vi "BuildUI.vi"(8 "error in (no error)":errorcluster, 11 "reference in":refnum<class "ProjectBuilder.lvclass">) -> (0 "error out":errorcluster, 3 "reference out":refnum<class "ProjectBuilder.lvclass">)   [LabVIEW 2015, in "ProjectBuilder.lvclass"]
uses:
  ProjectBuilder.lvclass
  BrowerTree/Type Definition/Symbol Index.ctl
  Product/Interface/Type Definition/BuildUI Workflow.ctl
  ProjectBuilder.lvclass/ProjectBuilder.ctl
  <vilib>/Utility/error.llb/Error Cluster From Error Code.vi
  <vilib>/ErrorRing/Error Ring.xnode
  Product/Interface/Part.lvclass
  AbstractBuilder/AbstractBuilder.lvclass
  BrowerTree/BrowerTree.lvclass
panel:
  in  "Previous":bool
  in  "Next":bool
  in  "Cancel":bool
  in  "SymbolIndex":T1
  in  "ComponentName":string caption="Name"
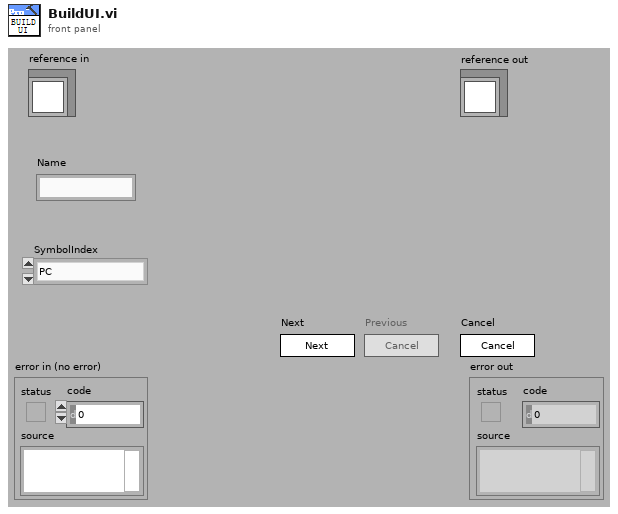
[diagram p1: front panel]
types:
  T1 = typedef "BrowerTree.lvclass/Symbol Index.ctl" = enum16{"PC", "Project", "Module", "DebugTask", "Communication"}
  T2 = typedef "AbstractBuilder.lvclass/BuildUI Workflow.ctl" = enum16{"Init", "Work", "Finish"}
  T3 = enum8{"Enabled", "Disabled", "Disabled and Grayed Out"}
  T4 = enum32{"Invalid", "Standard", "Closed", "Hidden", "Minimized", "Maximized"}
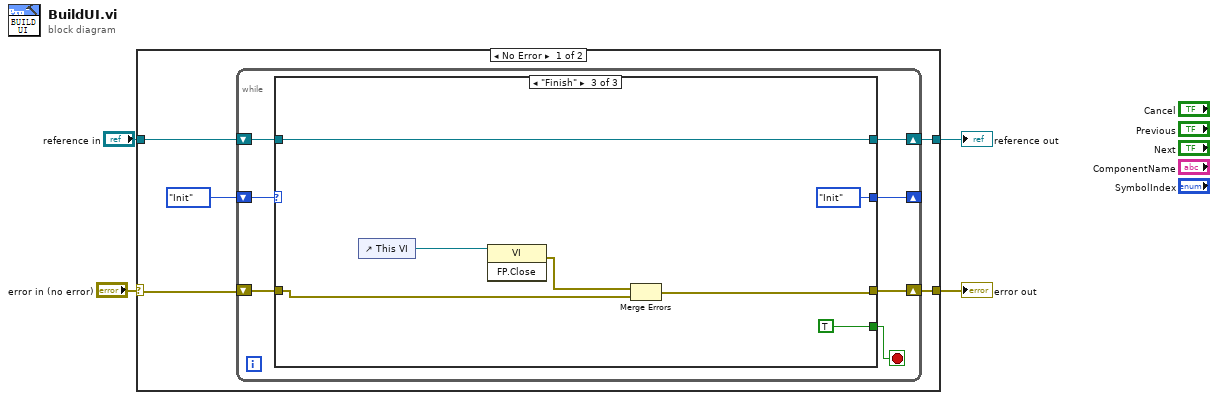
[diagram p0: block diagram]
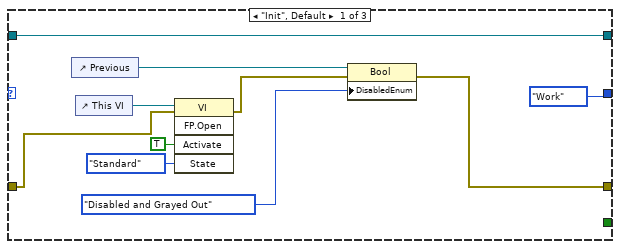
[diagram p2: hidden frame]
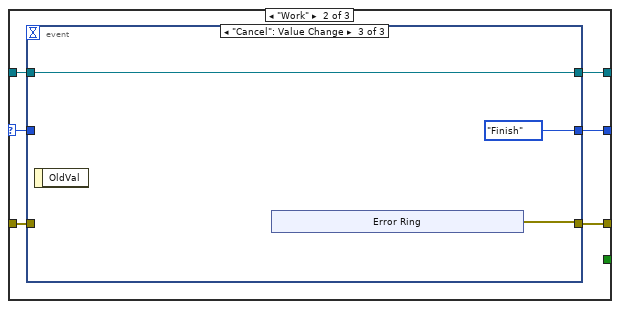
[diagram p3: hidden frame]
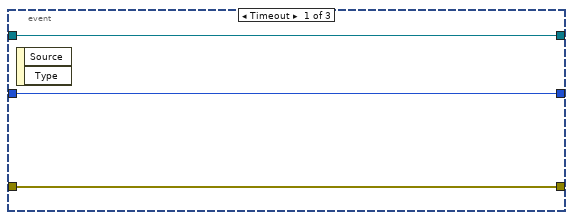
[diagram p4: hidden frame]
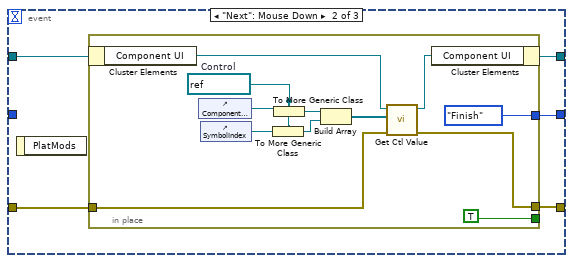
[diagram p5: hidden frame]
diagram:
  n1 = case shown="No Error" "error in (no error)" {
    selector: "error in (no error)" -> [w5 w69]
    tunnel: [w7 w69] -> w3
    tunnel: [w8 w68] -> w1
    tunnel: "reference in" -> [w9 w68]
    frame No Error {
      n2 = while {
        shift-right: [w13] -> w7
        shift-left: w5 -> [w16]
        shift-right: [w11] -> _
        shift-left: BuildUI_Workflow."Init" -> [w12]
        shift-right: [w14] -> w8
        shift-left: w9 -> [w15]
        stop <- w10 stop-if-true
        n3 = case shown="\"Finish\"" w12 {
          selector: w12 -> [_ w27 _]
          tunnel: w16 -> [w23 w32 w62]
          tunnel: w15 -> [w18 w31 w67]
          tunnel: [w18 w30 w67] -> w14
          tunnel: [w19 w29 w61] -> w13
          tunnel: [BuildUI_Workflow."Work" w28 BuildUI_Workflow."Init"] -> w11
          tunnel: [_ _ TRUE] -> w10
          frame "Init", Default {
            n4 = control-ref of="Previous"() -> (w22:refnum<vi>)
            n5 = control-ref of="This VI"() -> (w26:refnum<vi>)
            n6 = invoke class="VI" method="FP.Open"(reference=w26, error in=w23, "Activate"=TRUE ("Activate?"), "State"=T4."Standard") -> (error out=w20:errorcluster)  [unwired: 1 in, 4 out]
            n7 = property class="Bool"(reference=w22, error in=w20, "DisabledEnum"=T3."Disabled and Grayed Out" ("Disabled")) -> (error out=w19:errorcluster)  [unwired: 1 out]
          }
          frame "Work" {
            n8 = event shown="[2] \"Cancel\": Value Change" {
              selector: _ -> [_ _ _]
              dyn-events: _ -> [_ _ _]
              timeout: _ -> [_ _ _]
              tunnel: w32 -> [w34 w40 _]
              tunnel: w31 -> [w35 w39 w55]
              tunnel: [w35 w38 w55] -> w30
              tunnel: [w34 w37 w53] -> w29
              tunnel: [w33 w36 BuildUI_Workflow."Finish"] -> w28
              tunnel: w27 -> [w33 _ _]
              event Timeout {
                n9 = event-data() -> ()  [unwired: 1 in, 2 out]
              }
              event "Next": Mouse Down {
                n10 = event-data() -> ()  [unwired: 1 in, 1 out]
                n11 = in-place {
                  in-place-border: w40 -> [w46]
                  in-place-border: [w43] -> w37
                  in-place-border: [TRUE] -> _
                  in-place-border: [BuildUI_Workflow."Finish"] -> w36
                  w50 = refnum<vi> refnum  # Control
                  n12 = in-place-cluster #1(w39) -> ("Component UI"=w45:refnum<class "Part.lvclass">)
                  n13 = control-ref of="ComponentName"() -> (w52:refnum<vi>)
                  n14 = control-ref of="SymbolIndex"() -> (w51:refnum<vi>)
                  n15 = To More Generic Class(target class=w50, reference=w51) -> (generic class reference=w48:refnum<vi>)
                  n16 = To More Generic Class(target class=w50, reference=w52) -> (generic class reference=w49:refnum<vi>)
                  n17 = Build Array(w49, w48) -> (w47:refnum<vi>[])
                  n18 = call "Get Ctl Value.vi"("error in (no error)"=w46, "Control Refs"=w47, "Part in"=w45) -> ("error out"=w43:errorcluster, "Part out"=w44:refnum<class "Part.lvclass">)  [unwired: 7 in]
                  n19 = in-place-cluster #1("Component UI"=w44) -> (w38:refnum<class "ProjectBuilder.lvclass">)
                }
              }
              event "Cancel": Value Change {
                n20 = event-data() -> ()  [unwired: 1 in, 1 out]
                n21 = xnode "Error Ring"() -> ("error out"=w53:errorcluster)
              }
            }
          }
          frame "Finish" {
            n22 = control-ref of="This VI"() -> (w64:refnum<vi>)
            n23 = invoke class="VI" method="FP.Close"(reference=w64) -> (error out=w63:errorcluster)  [unwired: 2 in, 2 out]
            n24 = Merge Errors(w63, w62) -> (w61:errorcluster)
          }
        }
      }
    }
    frame Error {
    }
  }
  "error out" <- w3
  "reference out" <- w1
